vi "to string.vi"(8 "error in":errorcluster, 11 "JSON_RPC_Interface configuration in":refnum<class "JSON_RPC_Interface configuration.lvclass">) -> (0 "error out":errorcluster, 1 "data":string, 2 "version":string, 3 "JSON_RPC_Interface configuration out":refnum<class "JSON_RPC_Interface configuration.lvclass">)   [LabVIEW 2017, in "JSON_RPC_Interface configuration.lvclass"]
doc: "Provides an interface for saving a module configuration to a file or other serialized data source. It is recommended that all children of this class store data in two sets--data required for its own initialization, and any data required for parent initialization--and that each implementation uses the <b>Call Parent Method</b> primitive to serialize parent information."
uses:
  JSON_RPC_Interface configuration.lvclass
  current version.vi
  <vilib>/NI/Tag Bus Module Framework/module configuration/TBM module configuration.lvclass
  <vilib>/NI/Configuration Framework/serializable configuration/NISE_CEF_serializable configuration.lvclass
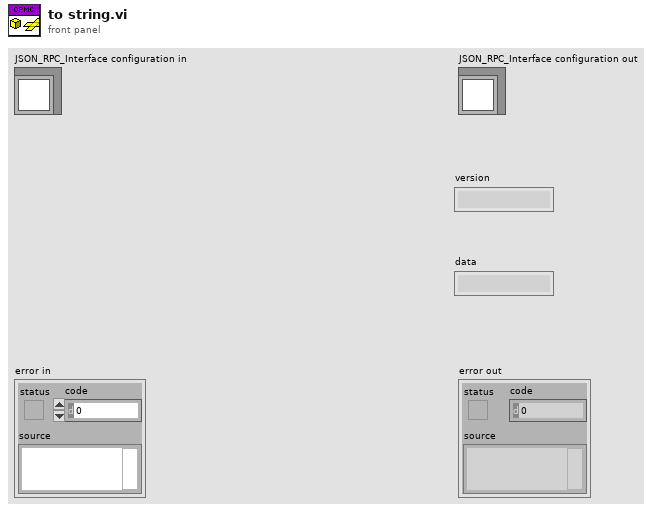
[diagram p1: front panel]
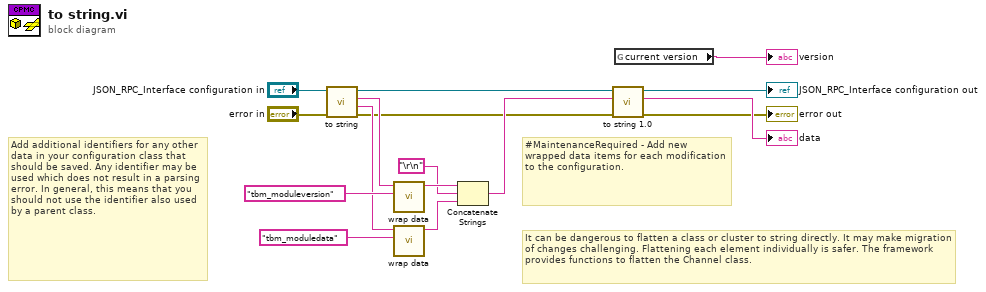
[diagram p0: block diagram]
diagram:
  # "#MaintenanceRequired - Add new wrapped data items for each modification to the configuration."
  # "It can be dangerous to flatten a class or cluster to string directly. It may make migration of changes challenging. Flattening each element individually is safer. The framework provides functions to flatten the Channel class."
  # "Add additional identifiers for any other data in your configuration class that should be saved. Any identifier may be used which does not result in a parsing error. In general, this means that you should not use the identifier also used by a parent class."
  n1 = call-parent "to string.vi"("error in"="error in", "module configuration in"="JSON_RPC_Interface configuration in") -> ("error out"=w2:errorcluster, "data"=w9:string, "version"=w10:string, "module configuration out"=w4:refnum<class "JSON_RPC_Interface configuration.lvclass">)  [unwired: 6 in]
  n2 = call <vilib>:"wrap data.vi"("identifier"="tbm_moduleversion" ("additional identifier"), "data to wrap"=w10) -> ("wrapped data"=w12:string)  [unwired: 9 in]
  n3 = call <vilib>:"wrap data.vi"("identifier"="tbm_moduledata" ("additional identifier"), "data to wrap"=w9) -> ("wrapped data"=w11:string)  [unwired: 9 in]
  n4 = Concatenate Strings(w12, "\r\n", w11) -> (w6:string)
  n5 = call "to string 1.0.vi"("error in (no error)"=w2, "data in"=w6, "JSON_RPC_Interface configuration in"=w4) -> ("error out"=→"error out":errorcluster, "data out"=→"data":string, "JSON_RPC_Interface configuration out"=→"JSON_RPC_Interface configuration out":refnum<class "JSON_RPC_Interface configuration.lvclass">)  [unwired: 6 in]
  n6 = global read "current version.vi" "current version"() -> (→"version":string)
